vi "Create Combination 3.vi"(6 "Element":i32, 7 "Combinations In":dbl[][](array[numeric]), 9 "Array":dbl[](array[numeric])=[1.0, 2.0, 3.0, 4.0, 5.0], 10 "Index":i32, 11 "Temp Combination":dbl[](array[numeric])) -> (4 "Element out":i32, 5 "Combinations Out":dbl[][](array[numeric]))   [LabVIEW 2018]
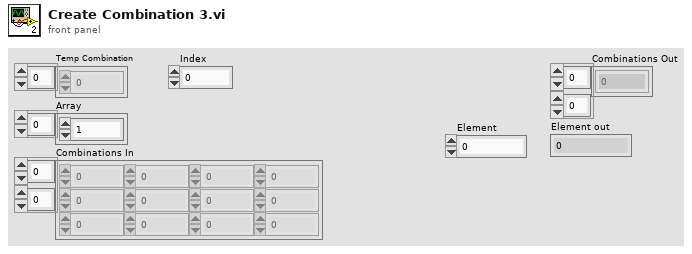
[diagram p1: front panel]
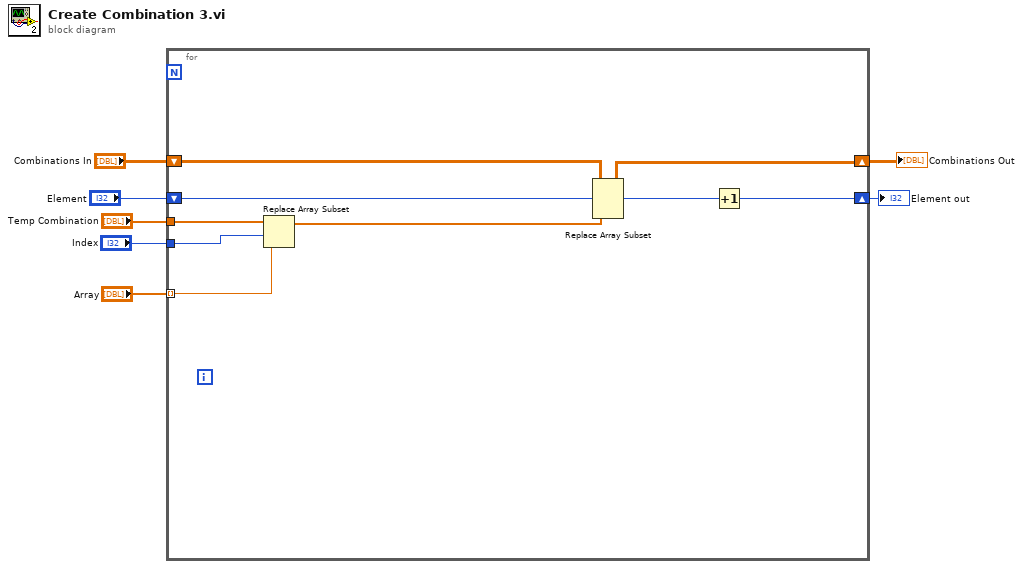
[diagram p0: block diagram]
diagram:
  n1 = for {
    tunnel: "Temp Combination" -> [w15]
    tunnel: "Array" -> [w14] mode=indexing
    tunnel: "Index" -> [w13]
    shift-right: [w11] -> w4
    shift-left: "Combinations In" -> [w12]
    shift-right: [w8] -> w1
    shift-left: "Element" -> [w9]
    n2 = Replace Array Subset(array=w15, new element=w14, index=w13) -> (w10:dbl[])
    n3 = Replace Array Subset(array=w12, new element=w10, index (row)=w9) -> (w11:dbl[][])  [unwired: 1 in]
    n4 = Increment(x=w9) -> (x+1=w8:i32)
  }
  "Combinations Out" <- w4
  "Element out" <- w1
